vi "InitVisPaths.vi"(8 "ErrorArray In":errorcluster[](array[cluster])) -> (0 "ErrorArray Out":errorcluster[](array[cluster]), 2 "VisualizeFilePaths":path[](array[path]))   [LabVIEW 2017, in "Framework.lvlib"]
uses:
  Framework.lvlib
  <userlib>/NIST/NISTErrorLib/NISTErrorLib.lvlib
panel:
  in  "Relative Path to Plugins":path=path "../../../Visualization/VisualizeApp_class"
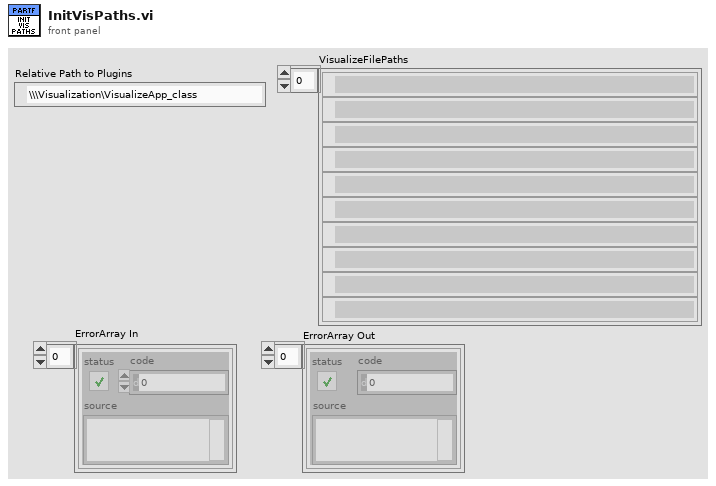
[diagram p1: front panel]
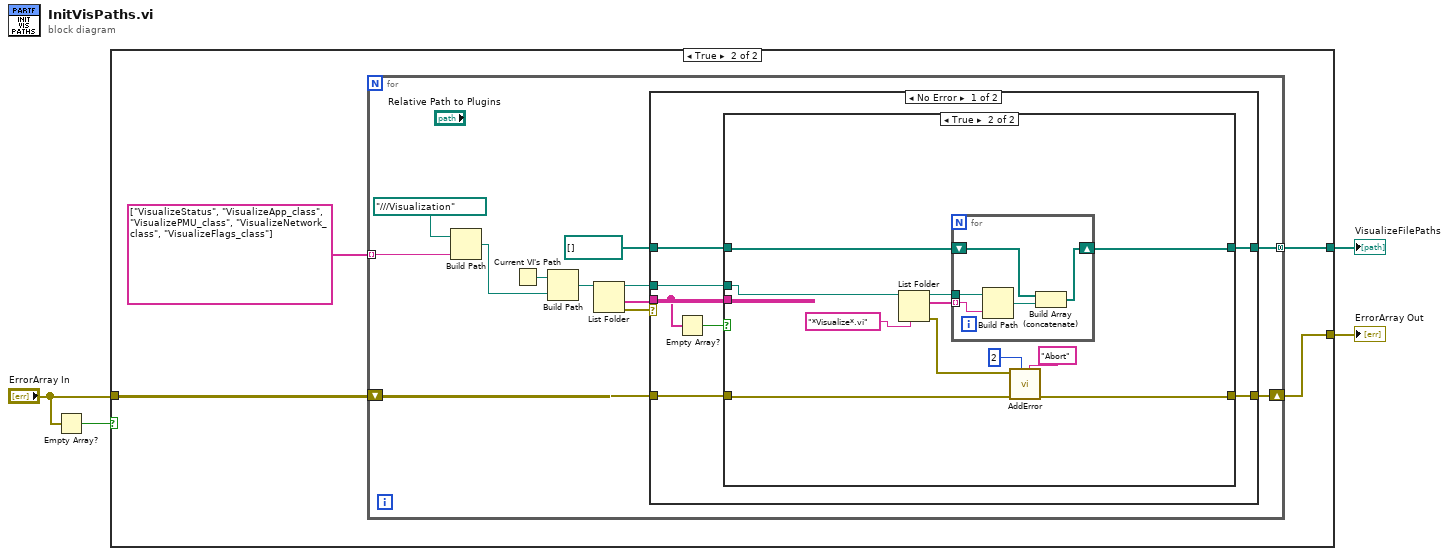
[diagram p0: block diagram]
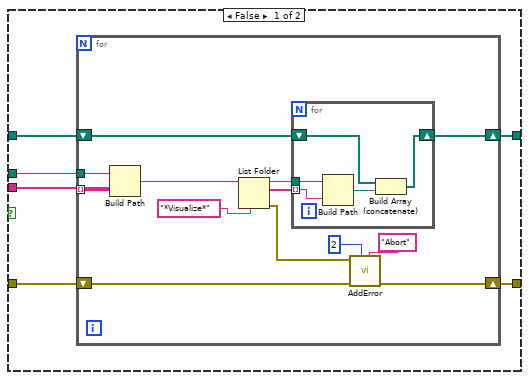
[diagram p3: hidden frame]
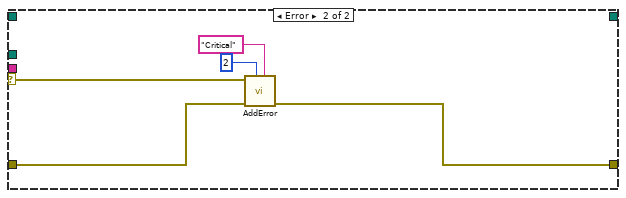
[diagram p4: hidden frame]
diagram:
  n1 = Empty Array?(array="ErrorArray In") -> (empty?=w4:bool)
  n2 = case shown="True" w4 {
    tunnel: "ErrorArray In" -> [w5 w9]
    tunnel: [w5 w6] -> w2
    tunnel: [_ w8] -> w1
    frame False {
    }
    frame True {
      n3 = for {
        tunnel: [w14] -> w8 mode=concatenating
        shift-right: [w10] -> w6
        shift-left: w9 -> [w18]
        tunnel: string[] ["VisualizeStatus", "VisualizeApp_class", "VisualizePMU_class", "VisualizeNetwork_class", "VisualizeFlags_class"] -> [w13] mode=indexing
        n4 = Build Path(base path=path "../../../Visualization", name or relative path=w13) -> (appended path=w11:path)
        n5 = Current VI's Path() -> (path=w21:path)
        n6 = Build Path(base path=w21, name or relative path=w11) -> (appended path=w20:path)
        n7 = List Folder(path=w20) -> (path out=w15:path, folder names=w16:string[], error out=w19:errorcluster)  [unwired: 3 in, 1 out]
        n8 = case shown="No Error" w19 {
          selector: w19 -> [_ w72]
          tunnel: w18 -> [w26 w73]
          tunnel: [w25 w69] -> w10
          tunnel: path[] [] ("EvtINIFilePaths 2") -> [w28 _]
          tunnel: w16 -> [w22 _]
          tunnel: w15 -> [w27 _]
          tunnel: [w24 _] -> w14
          frame No Error {
            n9 = Empty Array?(array=w22) -> (empty?=w23:bool)
            n10 = case shown="True" w23 {
              tunnel: w28 -> [w34 w56]
              tunnel: w22 -> [w33 _]
              tunnel: w27 -> [w32 w55]
              tunnel: w26 -> [w31 w57]
              tunnel: [w30 w53] -> w25
              tunnel: [w29 w54] -> w24
              frame False {
                n11 = for {
                  shift-right: [w40] -> w29
                  shift-left: w34 -> [w41]
                  tunnel: w33 -> [w43] mode=indexing
                  tunnel: w32 -> [w44]
                  shift-right: [w38] -> w30
                  shift-left: w31 -> [w39]
                  n12 = Build Path(base path=w44, name or relative path=w43) -> (appended path=w46:path)
                  n13 = List Folder(path=w46, pattern="*Visualize*") -> (path out=w42:path, filenames=w45:string[], error out=w35:errorcluster)  [unwired: 2 in, 1 out]
                  n14 = for {
                    tunnel: w45 -> [w50] mode=indexing
                    tunnel: w42 -> [w51]
                    shift-right: [w49] -> w40
                    shift-left: w41 -> [w48]
                    n15 = Build Path(base path=w51, name or relative path=w50) -> (appended path=w52:path)
                    n16 = Build Array (concatenate)(w48, w52) -> (w49:path[])
                  }
                  n17 = call <userlib>:"AddError.vi"("Severity"="Abort", "Priority"=u8 2, "ErrorArray"=w39, "error in (no error)"=w35) -> ("ErrorArray"=w38:errorcluster[])  [unwired: 6 in, 1 out]
                }
              }
              frame True {
                n18 = List Folder(path=w55, pattern="*Visualize*.vi") -> (path out=w61:path, filenames=w62:string[], error out=w58:errorcluster)  [unwired: 2 in, 1 out]
                n19 = for {
                  tunnel: w62 -> [w66] mode=indexing
                  tunnel: w61 -> [w67]
                  shift-right: [w65] -> w54
                  shift-left: w56 -> [w64]
                  n20 = Build Path(base path=w67, name or relative path=w66) -> (appended path=w68:path)
                  n21 = Build Array (concatenate)(w64, w68) -> (w65:path[])
                }
                n22 = call <userlib>:"AddError.vi"("Severity"="Abort", "Priority"=u8 2, "ErrorArray"=w57, "error in (no error)"=w58) -> ("ErrorArray"=w53:errorcluster[])  [unwired: 6 in, 1 out]
              }
            }
          }
          frame Error {
            n23 = call <userlib>:"AddError.vi"("Severity"="Critical", "Priority"=u8 2, "ErrorArray"=w73, "error in (no error)"=w72) -> ("ErrorArray"=w69:errorcluster[])  [unwired: 6 in, 1 out]
          }
        }
      }
    }
  }
  "ErrorArray Out" <- w2
  "VisualizeFilePaths" <- w1
